vi "Recording Path.vi"(8 "error in (no error)":errorcluster, 11 "TimeStamper in":refnum<class "TimeStamper.lvclass">) -> (0 "error out":errorcluster, 2 "FilePath":path, 3 "TimeStamper out":refnum<class "TimeStamper.lvclass">)   [LabVIEW 2014, in "TimeStamper.lvclass"]
uses:
  TimeStamper.lvclass
  <vilib>/Utility/config.llb/Read Key (Path).vi
  <vilib>/Utility/config.llb/NI_LVConfig.lvlib
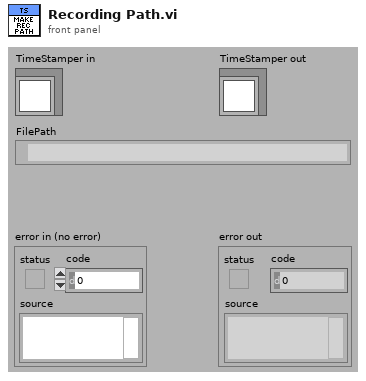
[diagram p1: front panel]
types:
  T1 = typedef "NI_LVConfig.lvlib/Config Data RefNum.ctl" = refnum<k1>
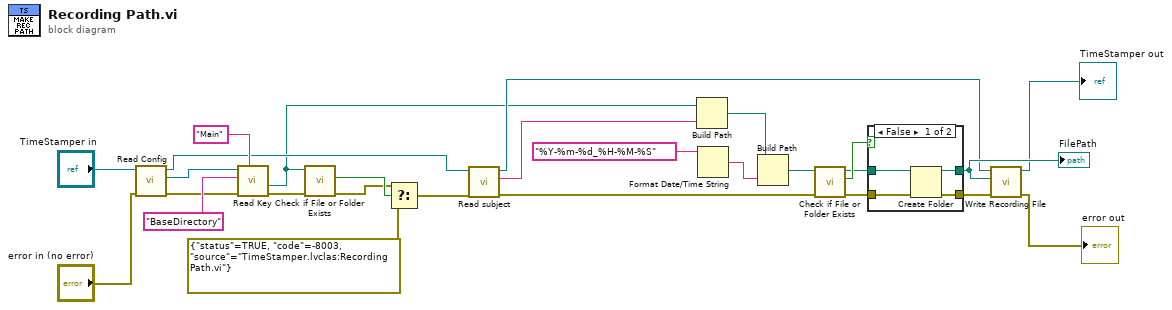
[diagram p0: block diagram]
diagram:
  n1 = call-dynamic "Read Config.vi"("error in (no error)"="error in (no error)", "AcquistionObject in"="TimeStamper in") -> ("error out"=w7:errorcluster, "config data"=w14:T1, "AcquistionObject out"=w9:refnum<class "TimeStamper.lvclass">)  [unwired: 7 in]
  n2 = call-poly <vilib>:"Read Key.vi"("section"="Main", "error in (no error)"=w7, "key"="BaseDirectory", "refnum"=w14) -> ("error out"=w3:errorcluster, "value"=w6:path)  [unwired: 4 in, 2 out]
  n3 = call <vilib>:"Check if File or Folder Exists.vi"("error in (no error)"=w3, "path"=w6) -> ("error out"=w1:errorcluster, "file or folder exists?"=w5:bool)  [unwired: 8 out]
  n4 = Select(t=w1, s=w5, f=errorcluster {"status"=TRUE, "code"=-8003, "source"="TimeStamper.lvclas:Recording Path.vi"} ("t")) -> (s? t:f=w2:errorcluster)
  n5 = call-dynamic "Read subject.vi"("error in (no error)"=w2, "TimeStamper in"=w9) -> ("error out"=w20:errorcluster, "subject"=w22:string, "TimeStamper out"=w11:refnum<class "TimeStamper.lvclass">)  [unwired: 7 in]
  n6 = Build Path(base path=w6, name or relative path=w22) -> (appended path=w27:path)
  n7 = Format Date/Time String(time format string (%c)="%Y-%m-%d_%H-%M-%S") -> (date/time string=w24:string)  [unwired: 2 out]
  n8 = Build Path(base path=w27, name or relative path=w24) -> (appended path=w23:path)
  n9 = call <vilib>:"Check if File or Folder Exists.vi"("error in (no error)"=w20, "path"=w23) -> ("error out"=w18:errorcluster, "file or folder exists?"=w26:bool, "dup path"=w21:path)  [unwired: 7 out]
  n10 = case shown="False" w26 {
    tunnel: w21 -> [w31 w33]
    tunnel: [w30 w33] -> w16
    tunnel: w18 -> [w29 w32]
    tunnel: [w28 w32] -> w19
    frame False {
      n11 = Create Folder(path (use dialog)=w31, error in=w29) -> (created path=w30:path, error out=w28:errorcluster)  [unwired: 1 in, 1 out]
    }
    frame True {
    }
  }
  "FilePath" <- w16
  n12 = call-dynamic "Write Recording File.vi"("error in (no error)"=w19, "Recording File"=w16, "AcquistionObject in"=w11) -> ("error out"=→"error out":errorcluster, "AcquistionObject out"=→"TimeStamper out":refnum<class "TimeStamper.lvclass">)  [unwired: 7 in]
